vi "Training_model_2.vi"() -> ()   [LabVIEW 2018]
uses:
  <vilib>/Utility/file.llb/Read Delimited Spreadsheet (DBL).vi
panel:
  in  "Tab Control":enum32{"Page 1", "Page 2"}(tab)
  in  "stop":bool
  in  "Training Button":bool
  in  "Model Selector":ext(ring) items=["Linear", "MLP"]
  out "String for python function":string
  out "Array":dbl[](array[numeric])
  out "String":string
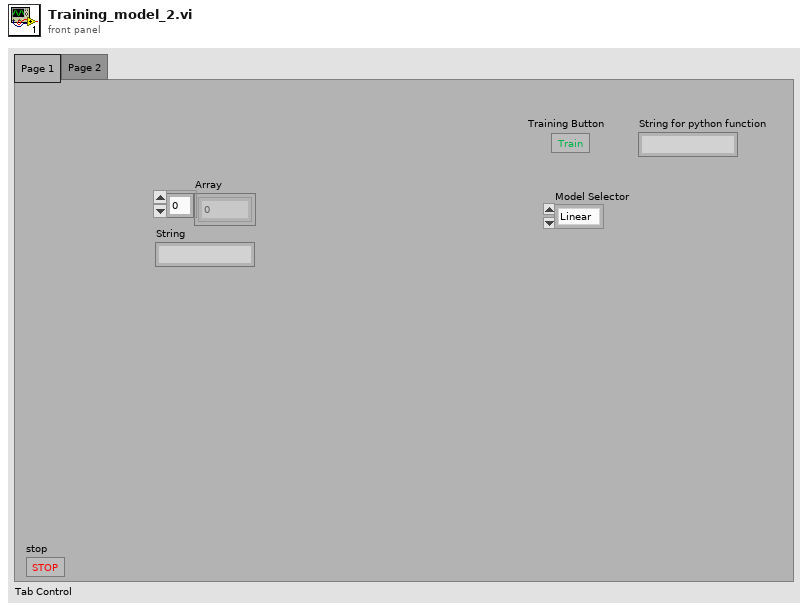
[diagram p1: front panel]
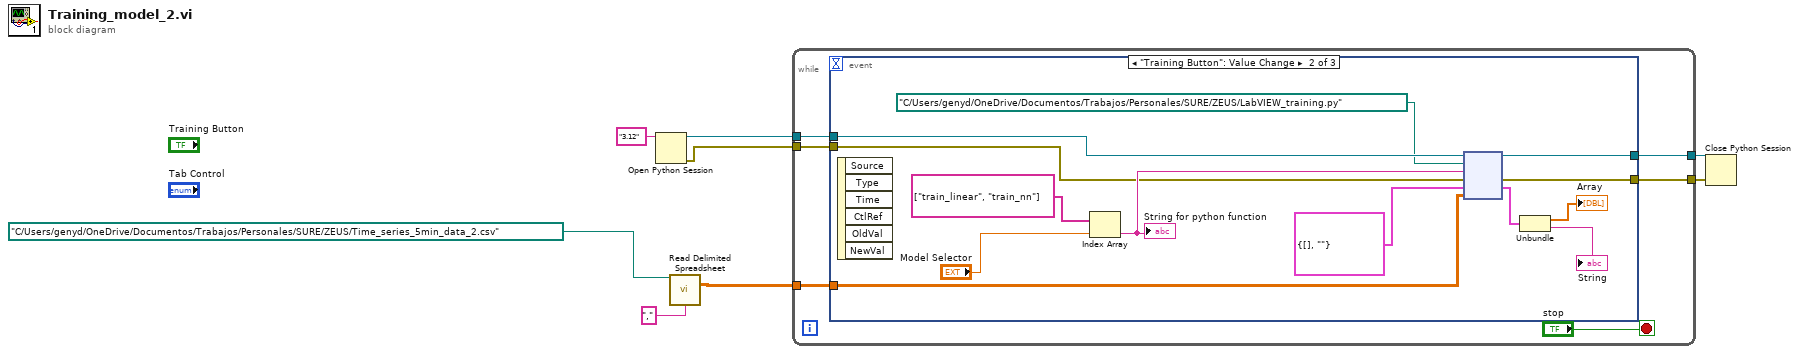
[diagram p0: block diagram]
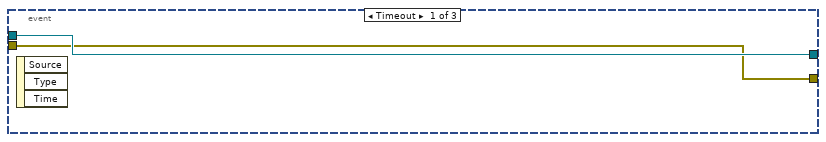
[diagram p2: hidden frame]
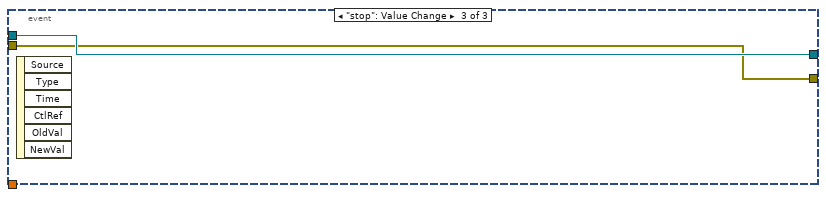
[diagram p3: hidden frame]
diagram:
  n1 = Open Python Session(python version="3.12" ("Python version")) -> (session out=w6:refnum<k35>, error out=w5:errorcluster)  [unwired: 2 in]
  n2 = call-poly <vilib>:"Read Delimited Spreadsheet.vi"("file path (dialog if empty)"=path "C:/Users/genyd/OneDrive/Documentos/Trabajos/Personales/SURE/ZEUS/Time_series_5min_data_2.csv", "delimiter (\\t)"="," ("delimiter (\\t)")) -> ("all rows"=w2:dbl[][])  [unwired: 8 in, 5 out]
  n3 = while {
    tunnel: w6 -> [w13]
    tunnel: w5 -> [w12]
    tunnel: [w11] -> w4
    tunnel: [w10] -> w3
    tunnel: w2 -> [w9]
    stop <- "stop" stop-if-true
    n4 = event shown="[1] \"Training Button\": Value Change" {
      selector: _ -> [_ _ _]
      dyn-events: _ -> [_ _ _]
      timeout: _ -> [_ _ _]
      tunnel: w13 -> [w16 w26 w31]
      tunnel: w12 -> [w15 w25 w30]
      tunnel: [w16 w24 w31] -> w11
      tunnel: [w15 w23 w30] -> w10
      tunnel: w9 -> [_ w22 _]
      event Timeout {
        n5 = event-data() -> ()  [unwired: 1 in, 3 out]
      }
      event "Training Button": Value Change {
        n6 = event-data() -> ()  [unwired: 1 in, 6 out]
        n7 = Index Array(array=string[] ["train_linear", "train_nn"], index="Model Selector") -> (element=w27:string)
        "String for python function" <- w27
        n8 = node(w26, path "C:/Users/genyd/OneDrive/Documentos/Trabajos/Personales/SURE/ZEUS/LabVIEW_training.py" ("module path"), w27, w25, cluster{dbl[], string} {[], ""}, w22) -> (w24:refnum<k35>, w23:errorcluster, w20:cluster{dbl[], string})  [unwired: 1 in, 2 out]
        n9 = Unbundle(w20) -> (→"Array":dbl[], →"String":string)
      }
      event "stop": Value Change {
        n10 = event-data() -> ()  [unwired: 1 in, 6 out]
      }
    }
  }
  n11 = Close Python Session(session in=w4, error in=w3) -> ()  [unwired: 1 out]
